vi "DAQmx_AO_test.vi"() -> ()   [LabVIEW 2020]
uses:
  Realization/NI Analog Output/NI Analog Output.lvclass
  Realization/NI DAQmx Base/TypeDefs/Channel Config.ctl
  Realization/NI DAQmx Base/NI DAQmx Base.lvclass
  Realization/NI Analog Output/TypeDefs/Timing Config.ctl
  Realization/NI Analog Output/TypeDefs/Trigger Config.ctl
panel:
  out "self-cal":variant
  out "self-test":variant
  out "error out":errorcluster
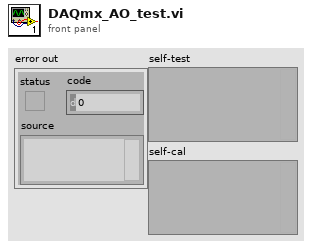
[diagram p1: front panel]
types:
  T1 = typedef "NI DAQmx.lvlib/NI DAQmx Base.lvclass/Channel Config.ctl" = cluster{"channels":string, "maximum value":dbl, "minimum value":dbl, "output terminal configuration":i32, "units":i32}
  T2 = typedef "NI DAQmx.lvlib/NI Analog Output.lvclass/Trigger Config.ctl" = cluster{"trigger type":string, "source":string, "slope":i32, "analog level":dbl, "analog hysteresis":dbl}
  T3 = typedef "NI DAQmx.lvlib/NI Analog Output.lvclass/Timing Config.ctl" = cluster{"sample mode":i32, "samples per channel":i32, "rate":dbl, "source":string, "active edge":i32}
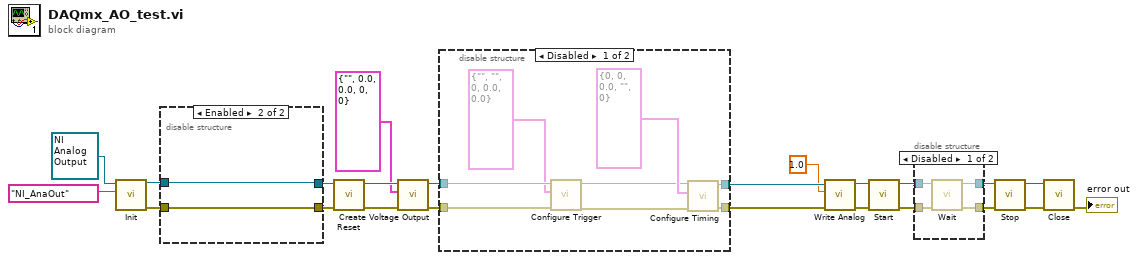
[diagram p0: block diagram]
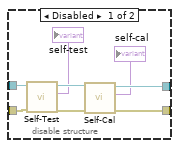
[diagram p4: hidden frame]
diagram:
  n1 = call-dynamic "Init.vi"("Params"="NI_AnaOut", "DAQmx Base in"=refnum<class "NI Analog Output.lvclass"> refnum ("NI DAQmx.lvlib:NI Analog Output.lvclass")) -> ("error out"=w23:errorcluster, "DAQmx Base out"=w22:refnum<class "NI Analog Output.lvclass">)  [unwired: 8 in]
  n2 = disable-structure shown="Enabled" {
    disable-tunnel: w23 -> [w31 w32]
    disable-tunnel: w22 -> [w30 w33]
    disable-tunnel: [w27 w33] -> w21
    disable-tunnel: [w26 w32] -> w20
    frame Disabled {
      n3 = call-dynamic "Self-Test.vi"("error in (no error)"=w31, "DAQmx Base in"=w30) -> ("error out"=w28:errorcluster, "Result"=→"self-test":variant, "DAQmx Base out"=w29:refnum<class "NI Analog Output.lvclass">)  [unwired: 7 in]
      n4 = call-dynamic "Self-Cal.vi"("error in (no error)"=w28, "DAQmx Base in"=w29) -> ("error out"=w26:errorcluster, "Result"=→"self-cal":variant, "DAQmx Base out"=w27:refnum<class "NI Analog Output.lvclass">)  [unwired: 7 in]
    }
    frame Enabled {
    }
  }
  n5 = call-dynamic "Reset.vi"("error in (no error)"=w20, "DAQmx Base in"=w21) -> ("error out"=w16:errorcluster, "DAQmx Base out"=w15:refnum<class "NI Analog Output.lvclass">)  [unwired: 8 in]
  n6 = call-dynamic "Create Voltage Output.vi"("error in (no error)"=w16, "Params"=T1 {"channels"="", "maximum value"=0.0, "minimum value"=0.0, "output terminal configuration"=0, "units"=0} ("Channel Config"), "NI Analog Output in"=w15) -> ("error out"=w3:errorcluster, "NI Analog Output out"=w2:refnum<class "NI Analog Output.lvclass">)  [unwired: 7 in]
  n7 = disable-structure shown="Disabled" {
    disable-tunnel: [w41 w42] -> w5
    disable-tunnel: [w40 w43] -> w4
    disable-tunnel: w3 -> [w38 w43]
    disable-tunnel: w2 -> [w37 w42]
    frame Disabled {
      n8 = call-dynamic "Configure Trigger.vi"("error in (no error)"=w38, "Params"=T2 {"trigger type"="", "source"="", "slope"=0, "analog level"=0.0, "analog hysteresis"=0.0} ("Cluster"), "NI DAQmx Base in"=w37) -> ("error out"=w35:errorcluster, "NI DAQmx Base out"=w36:refnum<class "NI Analog Output.lvclass">)  [unwired: 7 in]
      n9 = call-dynamic "Configure Timing.vi"("error in (no error)"=w35, "Params"=T3 {"sample mode"=0, "samples per channel"=0, "rate"=0.0, "source"="", "active edge"=0} ("Timing Config"), "NI DAQmx Base in"=w36) -> ("error out"=w40:errorcluster, "NI DAQmx Base out"=w41:refnum<class "NI Analog Output.lvclass">)  [unwired: 7 in]
    }
    frame Enabled {
    }
  }
  n10 = call-dynamic "Write Analog.vi"("error in (no error)"=w4, "Params"=1.0, "NI Analog Output in"=w5) -> ("error out"=w8:errorcluster, "NI Analog Output out"=w7:refnum<class "NI Analog Output.lvclass">)  [unwired: 7 in]
  n11 = call-dynamic "Start.vi"("error in (no error)"=w8, "NI DAQmx Base in"=w7) -> ("error out"=w10:errorcluster, "NI DAQmx Base out"=w12:refnum<class "NI Analog Output.lvclass">)  [unwired: 8 in]
  n12 = disable-structure shown="Disabled" {
    disable-tunnel: w12 -> [w47 w49]
    disable-tunnel: [w46 w49] -> w11
    disable-tunnel: w10 -> [w45 w48]
    disable-tunnel: [w44 w48] -> w9
    frame Disabled {
      n13 = call-dynamic "Wait.vi"("error in (no error)"=w45, "NI DAQmx Base in"=w47) -> ("error out"=w44:errorcluster, "NI DAQmx Base out"=w46:refnum<class "NI Analog Output.lvclass">)  [unwired: 8 in]
    }
    frame Enabled {
    }
  }
  n14 = call-dynamic "Stop.vi"("error in (no error)"=w9, "NI DAQmx Base in"=w11) -> ("error out"=w13:errorcluster, "NI DAQmx Base out"=w14:refnum<class "NI Analog Output.lvclass">)  [unwired: 8 in]
  n15 = call-dynamic "Close.vi"("error in (no error)"=w13, "DAQmx Base in"=w14) -> ("error out"=→"error out":errorcluster)  [unwired: 8 in, 1 out]
